vi "View.vi"(8 "error in (no error)":errorcluster, 10 "Debugger":refnum<class "Debug Process.lvclass">, 11 "Messages Composite View In":refnum<class "Messages Composite View.lvclass">) -> (0 "error out":errorcluster, 3 "Messages Composite View Out":refnum<class "Messages Composite View.lvclass">)   [LabVIEW 2020, in "Messages Composite View.lvclass"]
uses:
  Messages Composite View.lvclass
  C:/Users/anton/Documents/GitHub/triarc-debugger/source/Debug View/Debug View.lvclass
  Process/Debug Process.lvclass
  Debugger/Debugger.lvclass
  Debug View/Debug View.lvclass/Debug View.ctl
  Messages Composite View.lvclass/Messages Composite View.ctl
  Debug View/Debug View.lvclass
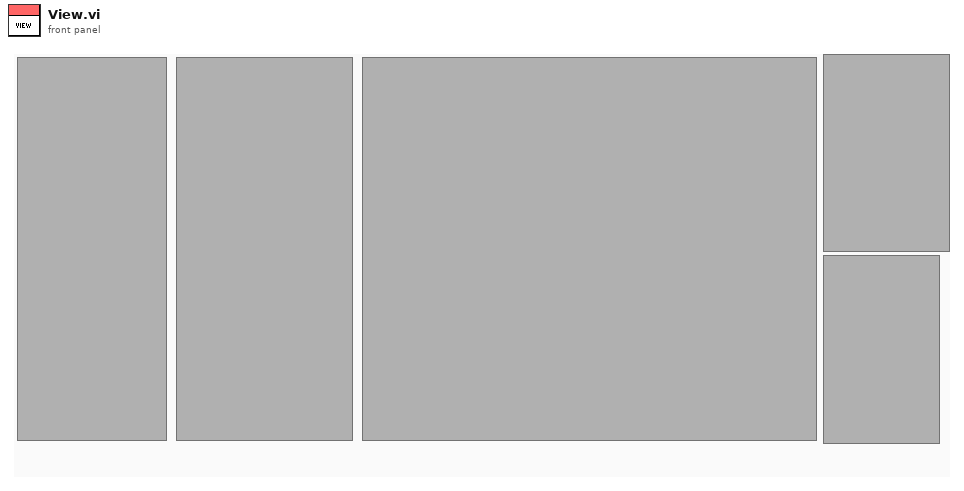
[diagram p1: front panel]
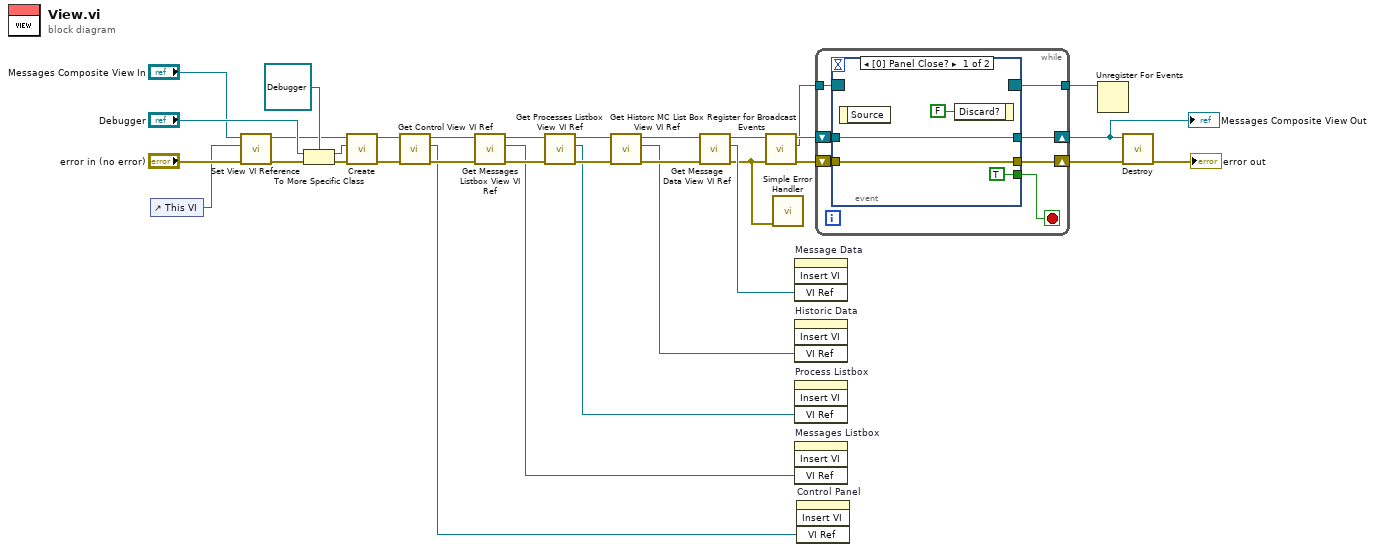
[diagram p0: block diagram]
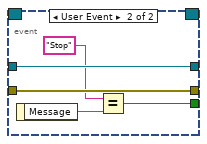
[diagram p2: hidden frame]
diagram:
  n1 = control-ref of="This VI"() -> (w2:refnum<vi>)
  n2 = call "Set View VI Reference.vi"("error in (no error)"="error in (no error)", "View VI ref"=w2, "Debug View in"="Messages Composite View In") -> ("error out"=w4:errorcluster, "Debug View out"=w5:refnum<class "Messages Composite View.lvclass">)  [unwired: 7 in]
  n3 = To More Specific Class(target class=refnum<class "Debugger.lvclass"> refnum ("Debugger"), reference="Debugger", error in=w4) -> (specific class reference=w14:refnum<class "Debugger.lvclass">, error out=w16:errorcluster)
  n4 = call "Create.vi"("error in (no error)"=w16, "Debugger"=w14, "Messages Composite View In"=w5) -> ("error out"=w19:errorcluster, "Messages Composite View Out"=w18:refnum<class "Messages Composite View.lvclass">)  [unwired: 7 in]
  n5 = call "Get Control View VI Ref.vi"("error in (no error)"=w19, "Messages Composite View In"=w18) -> ("error out"=w23:errorcluster, "VI Ref"=w21:refnum<vi>, "Messages Composite View Out"=w22:refnum<class "Messages Composite View.lvclass">)  [unwired: 7 in]
  n6 = call "Get Messages Listbox View VI Ref.vi"("error in (no error)"=w23, "Messages Composite View In"=w22) -> ("error out"=w31:errorcluster, "VI Ref"=w29:refnum<vi>, "Messages Composite View Out"=w30:refnum<class "Messages Composite View.lvclass">)  [unwired: 7 in]
  n7 = call "Get Processes Listbox View VI Ref.vi"("error in (no error)"=w31, "Messages Composite View In"=w30) -> ("error out"=w33:errorcluster, "VI Ref"=w32:refnum<vi>, "Messages Composite View Out"=w27:refnum<class "Messages Composite View.lvclass">)  [unwired: 7 in]
  n8 = call "Get Historc MC List Box View VI Ref.vi"("error in (no error)"=w33, "Messages Composite View In"=w27) -> ("error out"=w28:errorcluster, "VI Ref"=w26:refnum<vi>, "Messages Composite View Out"=w25:refnum<class "Messages Composite View.lvclass">)  [unwired: 7 in]
  n9 = call "Get Message Data View VI Ref.vi"("error in (no error)"=w28, "Messages Composite View In"=w25) -> ("error out"=w1:errorcluster, "VI Ref"=w24:refnum<vi>, "Messages Composite View Out"=w12:refnum<class "Messages Composite View.lvclass">)  [unwired: 7 in]
  n10 = call "Register for Broadcast Events.vi"("error in (no error)"=w1, "Process In"=w12) -> ("error out"=w13:errorcluster, "Event Registration Refnum Out"=w10:refnum<event-registration>, "Process Out"=w11:refnum<class "Messages Composite View.lvclass">)  [unwired: 7 in]
  n11 = call <vilib>:"Simple Error Handler.vi"("error in (no error)"=w1) -> ()  [unwired: 4 in, 5 out]
  n12 = invoke on="Message Data" class="SubPnl" method="Insert VI"("VI Ref"=w24) -> ()  [unwired: 3 in, 4 out]
  n13 = invoke on="Historic Data" class="SubPnl" method="Insert VI"("VI Ref"=w26) -> ()  [unwired: 3 in, 4 out]
  n14 = invoke on="Process Listbox" class="SubPnl" method="Insert VI"("VI Ref"=w32) -> ()  [unwired: 3 in, 4 out]
  n15 = invoke on="Messages Listbox" class="SubPnl" method="Insert VI"("VI Ref"=w29) -> ()  [unwired: 3 in, 4 out]
  n16 = invoke on="Control Panel" class="SubPnl" method="Insert VI"("VI Ref"=w21) -> ()  [unwired: 3 in, 4 out]
  n17 = while {
    tunnel: w10 -> [w36]
    shift-right: [w40] -> w20
    shift-left: w13 -> [w38]
    shift-right: [w39] -> w7
    shift-left: w11 -> [w37]
    tunnel: [w34] -> w9
    stop <- w35 stop-if-true
    n18 = event shown="[0] Panel Close?" {
      selector: w36 -> [_ _]
      dyn-events: [_ _] -> w34
      timeout: _ -> [_ _]
      tunnel: w38 -> [w43 w48]
      tunnel: w37 -> [w42 w49]
      tunnel: [w43 w48] -> w40
      tunnel: [w42 w49] -> w39
      tunnel: [TRUE w45] -> w35
      event Panel Close? {
        n19 = event-data() -> ()  [unwired: 1 in, 1 out]
        n20 = event-data("Discard?"=FALSE) -> ()  [unwired: 1 in, 1 out]
      }
      event User Event {
        n21 = event-data() -> ("Message"=w47:string)  [unwired: 1 in]
        n22 = Equal?(x="Stop", y=w47) -> (x = y?=w45:bool)
      }
    }
  }
  "Messages Composite View Out" <- w7
  n23 = Unregister For Events(event registration refnum=w9) -> ()  [unwired: 1 in, 1 out]
  n24 = call "Destroy.vi"("error in (no error)"=w20, "Messages Composite View In"=w7) -> ("error out"=→"error out":errorcluster)  [unwired: 9 in]
